vi "Serialize.vi"(8 "error in (no error)":errorcluster, 11 "VIP Uninstall in":refnum<class "VIPM Update.lvclass">) -> (0 "error out":errorcluster, 2 "Text":string)   [LabVIEW 2014, in "VIPM Update.lvclass"]
uses:
  VIPM Update.lvclass
  VIPM Update - STYP.ctl
  VIPM Update.lvclass/VIPM Update.ctl
  Read LV Version.vi
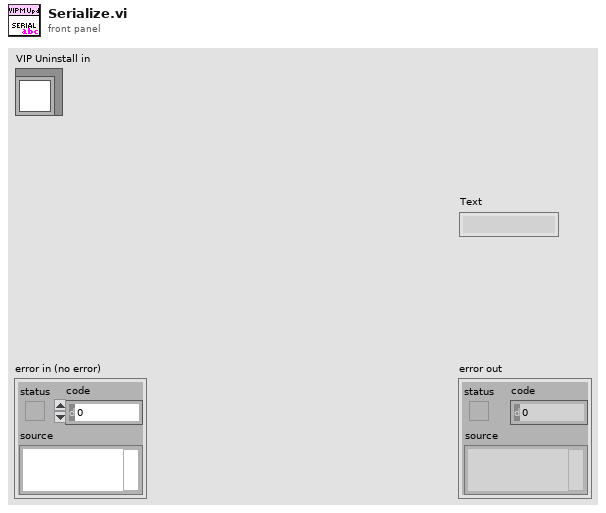
[diagram p1: front panel]
types:
  T1 = typedef "VIPM Update - STYP.ctl" = cluster{"LabVIEW Version":string}
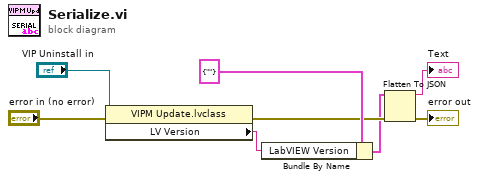
[diagram p0: block diagram]
diagram:
  n1 = property class="VIPM Update.lvclass"(reference="VIP Uninstall in", error in="error in (no error)") -> (error out=w4:errorcluster, "LV Version"=w5:string)  [unwired: 1 out]
  n2 = Bundle By Name(cluster=T1 {"LabVIEW Version"=""} ("VIPM Update"), "LabVIEW Version"=w5) -> (w2:T1)
  n3 = Flatten To JSON(anything=w2, error in (no error)=w4) -> (JSON string=→"Text":string, 11:→"error out":errorcluster)  [unwired: 1 in]
